vi "Configure Modulation (PWM).vi"(0 "VISA resource name":refnum<visa-resource-name>, 1 "Enable PWM (T: Enable)":bool=TRUE, 2 "Modulation Waveform (0: Sine)":u16(ring) items=["Sine", "Square", "Ramp", "Noise", "User Waveform", "Edit Memory", "EFile"], 5 "Channel (1 Channel 1)":u16(ring)=1 items=["Channel 1"=1, "Channel 2"=2], 7 "PWM Source (0: Internal)":u16(ring) items=["Internal", "External"], 9 "PWM Deviation (0%)":dbl, 11 "error in (no error)":errorcluster, 12 "Modulation Frequency (100.00 Hz)":dbl=100.0, 13 "User Waveform (0)":i32, 14 "EFile Name (\"\")":string) -> (4 "VISA resource name out":refnum<visa-resource-name>, 15 "error out":errorcluster)   [LabVIEW 2016, in "Tektronix AFG 1000 Series.lvlib"]
doc: "Configures and enables pulse width modulation (PWM).\n\n<b>Note:</b>\nThis VI is not supported for AFG1022."
uses:
  Tektronix AFG 1000 Series.lvlib
panel:
  # "Internal PWM Settings"
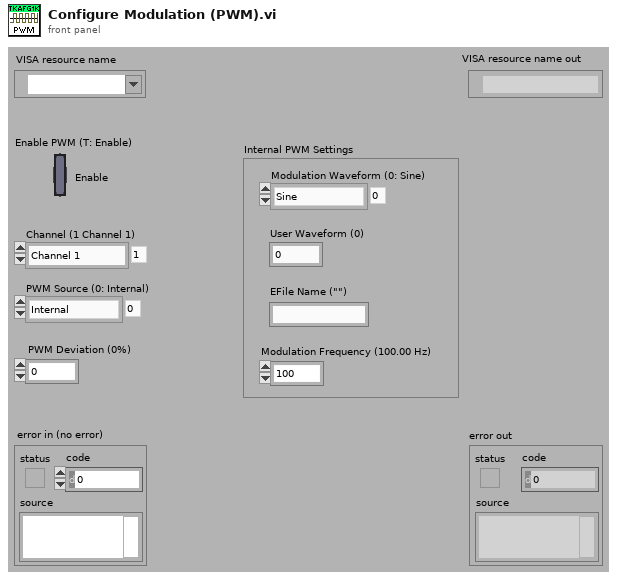
[diagram p1: front panel]
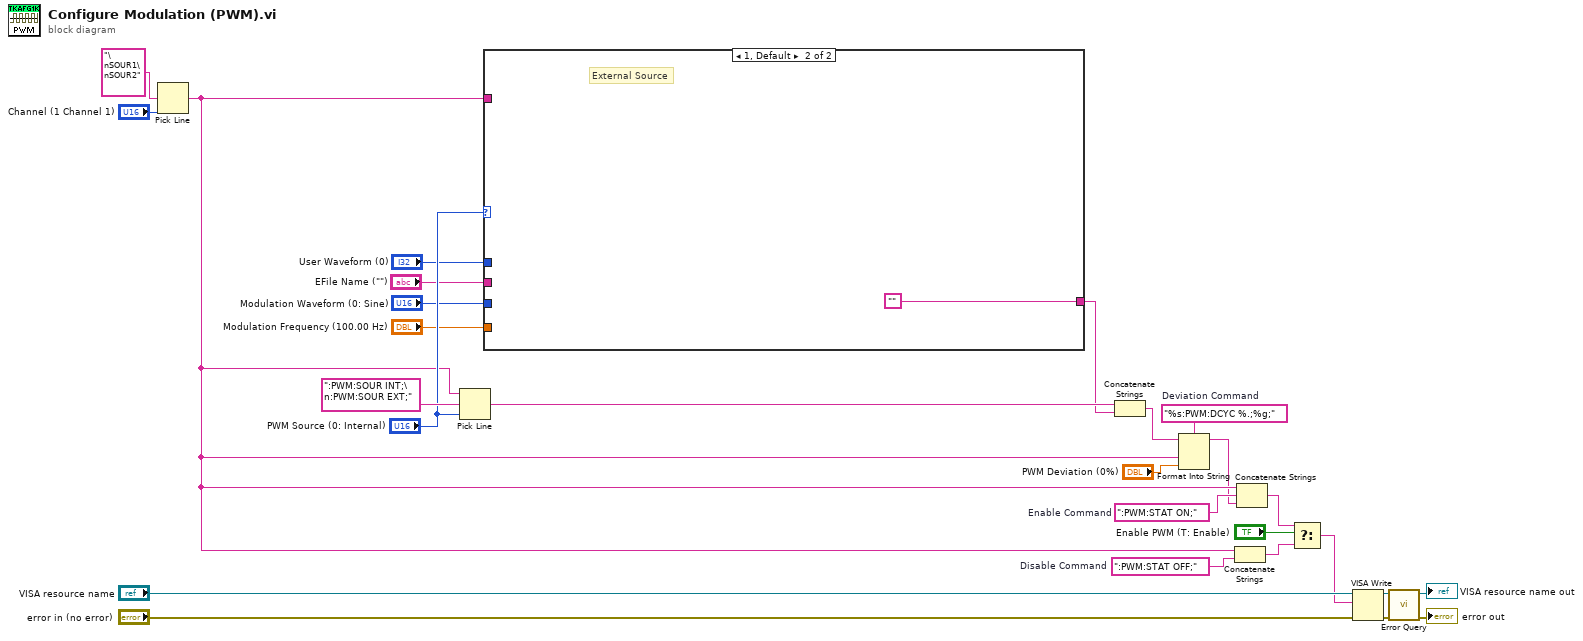
[diagram p0: block diagram]
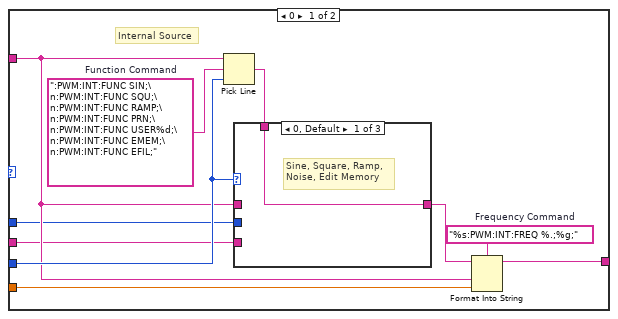
[diagram p2: hidden frame]
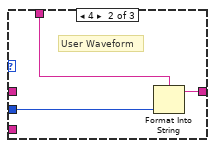
[diagram p3: hidden frame]
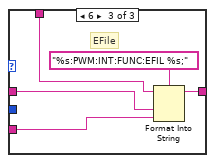
[diagram p4: hidden frame]
diagram:
  w19 = ":PWM:STAT ON;"  # Enable Command
  w21 = "%s:PWM:DCYC %.;%g;"  # Deviation Command
  w16 = ":PWM:STAT OFF;"  # Disable Command
  n1 = Pick Line(multi-line string="\nSOUR1\nSOUR2" ("string (\"\")"), line index="Channel (1 Channel 1)") -> (output string=w3:string)  [unwired: 1 in]
  n2 = Pick Line(string ("")=w3, multi-line string=":PWM:SOUR INT;\n:PWM:SOUR EXT;" ("Source Command"), line index="PWM Source (0: Internal)") -> (output string=w10:string)
  n3 = case shown="1, Default" "PWM Source (0: Internal)" {
    tunnel: w3 -> [w30 _]
    tunnel: [w35 ""] -> w4
    tunnel: "Modulation Waveform (0: Sine)" -> [w31 _]
    tunnel: "Modulation Frequency (100.00 Hz)" -> [w34 _]
    tunnel: "User Waveform (0)" -> [w29 _]
    tunnel: "EFile Name (\"\")" -> [w28 _]
    frame 0 {
      w36 = "%s:PWM:INT:FREQ %.;%g;"  # Frequency Command
      w37 = ":PWM:INT:FUNC SIN;\n:PWM:INT:FUNC SQU;\n:PWM:INT:FUNC RAMP;\n:PWM:INT:FUNC PRN;\n:PWM:INT:FUNC USER%d;\n:PWM:INT:FUNC EMEM;\n:PWM:INT:FUNC EFIL;"  # Function Command
      # "Internal Source"
      n4 = Pick Line(string ("")=w30, multi-line string=w37, line index=w31) -> (output string=w33:string)
      n5 = case shown="0, Default" w31 {
        tunnel: w33 -> [w38 w41 w45]
        tunnel: [w38 w40 w46] -> w32
        tunnel: w30 -> [_ _ w43]
        tunnel: w29 -> [_ w39 _]
        tunnel: w28 -> [_ _ w42]
        frame 0, Default {
          # "Sine, Square, Ramp,\nNoise, Edit Memory"
        }
        frame 4 {
          # "User Waveform"
          n6 = Format Into String(format string=w41, w39) -> (resulting string=w40:string)  [unwired: 2 in, 1 out]
        }
        frame 6 {
          # "EFile"
          n7 = Format Into String(format string="%s:PWM:INT:FUNC:EFIL %s;", initial string=w45, w43, w42) -> (resulting string=w46:string)  [unwired: 1 in, 1 out]
        }
      }
      n8 = Format Into String(format string=w36, initial string=w32, w30, w34) -> (resulting string=w35:string)  [unwired: 1 in, 1 out]
    }
    frame 1, Default {
      # "External Source"
    }
  }
  n9 = Concatenate Strings(w10, w4) -> (w9:string)
  n10 = Format Into String(format string=w21, initial string=w9, w3, "PWM Deviation (0%)") -> (resulting string=w1:string)  [unwired: 1 in, 1 out]
  n11 = Concatenate Strings(w3, w16) -> (w14:string)
  n12 = Concatenate Strings(w3, w19, w1) -> (w12:string)
  n13 = Select(t=w12, s="Enable PWM (T: Enable)", f=w14) -> (s? t:f=w13:string)
  n14 = VISA Write(VISA resource name="VISA resource name", write buffer=w13, error in (no error)="error in (no error)") -> (VISA resource name out=w24:refnum<visa-resource-name>, error out=w25:errorcluster)  [unwired: 1 out]
  n15 = call "Error Query.vi"("error in (no error)"=w25, "VISA resource name"=w24) -> ("error out"=→"error out":errorcluster, "VISA resource name out"=→"VISA resource name out":refnum<visa-resource-name>)  [unwired: 6 in, 2 out]
